vi "Save_to_Project.vi"(8 "error in (no error)":errorcluster, 9 "index in":string, 10 "buildObject":T2, 11 "IB_RegData_String in":refnum<class "IB_RegData_String.lvclass">) -> (0 "error out":errorcluster, 1 "index out":string, 2 "buildObject out":T2, 3 "IB_RegData_String out":refnum<class "IB_RegData_String.lvclass">)   [LabVIEW 2020, in "IB_RegData_String.lvclass"]
uses:
  <vilib>/AppBuilder/IB_Classes/RegData/RegData_String/IB_RegData_String.lvclass
  <vilib>/AppBuilder/IB_Classes/RegData/RegData_String/IB_RegData_String.lvclass/IB_RegData_String.ctl
  <vilib>/AppBuilder/IB_Classes/RegData/IB_RegData.lvclass
  <vilib>/AppBuilder/IB_RW_Project/IB_RW_Project_PropBag_Action.ctl
  <resource>/Framework/Providers/API/ItemRef.ctl
  <vilib>/AppBuilder/IB_RW_Project/IB_RW_Project_RegData_String_Data.ctl
panel:
  in  "RegData":T1
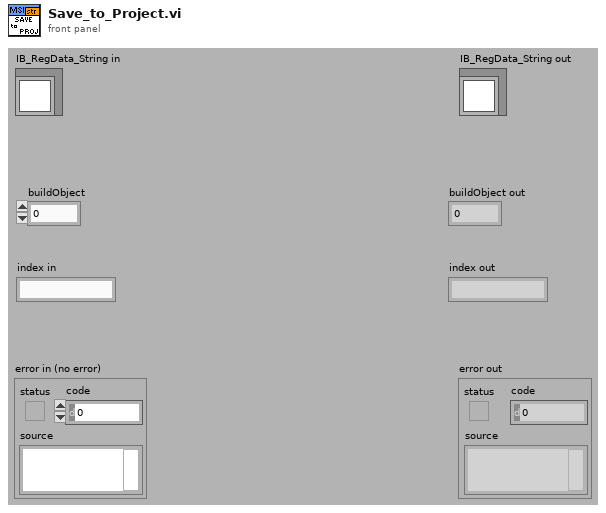
[diagram p1: front panel]
types:
  T1 = typedef "IB_RW_Project_RegData_String_Data.ctl" = cluster{"string":string}
  T2 = typedef "ItemRef.ctl" = u64
  T3 = typedef "IB_RW_Project_PropBag_Action.ctl" = enum16{"read", "write", "clear", "readPrevious", "writePrevious", "clearPrevious"}
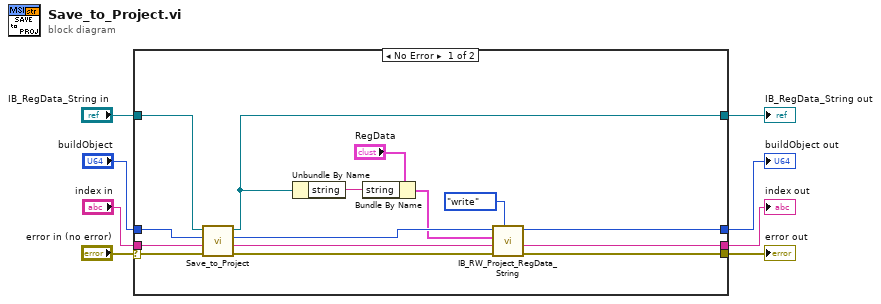
[diagram p0: block diagram]
diagram:
  n1 = case shown="No Error" "error in (no error)" {
    selector: "error in (no error)" -> [w20 w27]
    tunnel: [w14 w27] -> w8
    tunnel: [w12 w26] -> w7
    tunnel: [w10 w25] -> w6
    tunnel: [w18 w24] -> w5
    tunnel: "index in" -> [w23 w26]
    tunnel: "buildObject" -> [w22 w25]
    tunnel: "IB_RegData_String in" -> [w21 w24]
    frame No Error {
      n2 = call-parent "Save_to_Project.vi"("error in (no error)"=w20, "index in"=w23, "buildObject"=w22, "IB_RegData in"=w21) -> ("error out"=w15:errorcluster, "index out"=w13:string, "buildObject out"=w11:T2, "IB_RegData out"=w18:refnum<class "IB_RegData_String.lvclass">)  [unwired: 4 in]
      n3 = Unbundle By Name(w18) -> ("string"=w19:string)
      n4 = Bundle By Name(cluster="RegData", "string"=w19) -> (w9:T1)
      n5 = call <vilib>:"IB_RW_Project_RegData_String.vi"("action"=IB_RW_Project_PropBag_Action."write", "error in (no error)"=w15, "index in"=w13, "RegData"=w9, "buildObject"=w11) -> ("error out"=w14:errorcluster, "index out"=w12:string, "buildObject out"=w10:T2)  [unwired: 3 in, 1 out]
    }
    frame Error {
    }
  }
  "error out" <- w8
  "IB_RegData_String out" <- w5
  "buildObject out" <- w6
  "index out" <- w7
